vi "Tank Increment and Decrement Simulation.vi"() -> ()   [LabVIEW 2020]
panel:
  out "Tank":i32(slide) scale=0.0..100.0
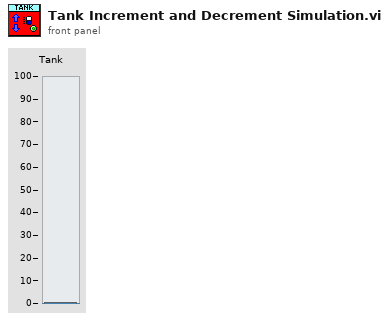
[diagram p1: front panel]
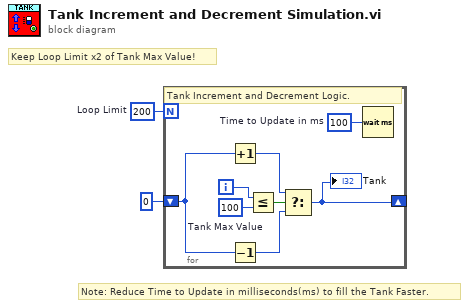
[diagram p0: block diagram]
diagram:
  w2 = 200  # Loop Limit
  # "Note: Reduce Time to Update in milliseconds(ms) to fill the Tank Faster."
  # "Keep Loop Limit x2 of Tank Max Value!"
  n1 = for {
    N: w2 -> [_]
    shift-right: [w3] -> _
    shift-left: 0 -> [w6]
    i -> [w10]
    w4 = u32 100  # Time to Update in ms
    w9 = 100  # Tank Max Value
    # "Tank Increment and Decrement Logic."
    n2 = Increment(x=w6) -> (x+1=w7:i32)
    n3 = Decrement(x=w6) -> (x-1=w5:i32)
    n4 = Less Or Equal?(x=w10, y=w9) -> (x <= y?=w8:bool)
    n5 = Select(t=w7, s=w8, f=w5) -> (s? t:f=w3:i32)
    "Tank" <- w3
    n6 = Wait (ms)(milliseconds to wait=w4) -> ()  [unwired: 1 out]
  }
